vi "HighlandTester.vi"() -> ()   [LabVIEW 2013]
uses:
  <vilib>/Instr/_visa.llb/VISA Configure Serial Port (Instr).vi
  AlicatPC/AlicatPC.lvclass
panel:
  out "PULSE":bool
  out "return count":u32
  out "read buffer":string
  out "auto queue commands response":string
  out "error out":errorcluster
  in  "command":string="TLEVEL 1.25; TLEVEL; TRIG POS"
  out "response":string
  in  "VISA resource name":refnum<visa-resource-name>
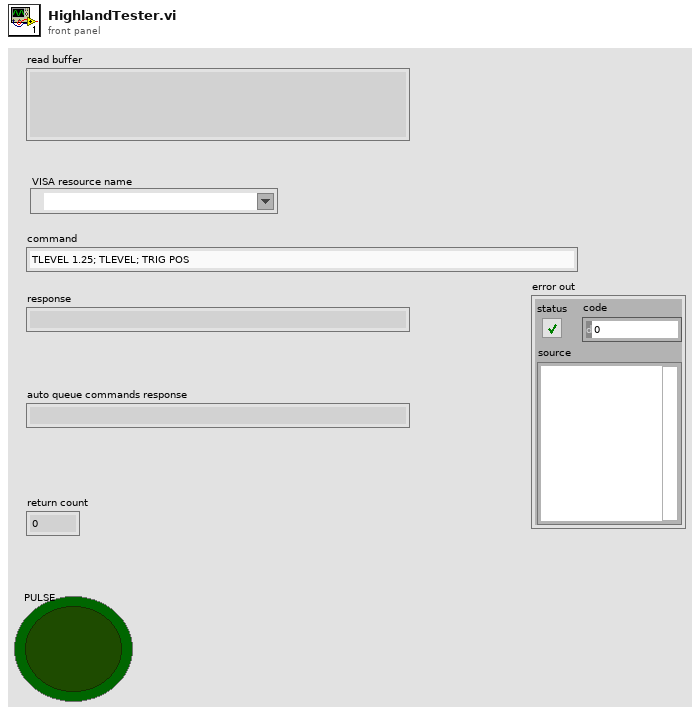
[diagram p1: front panel]
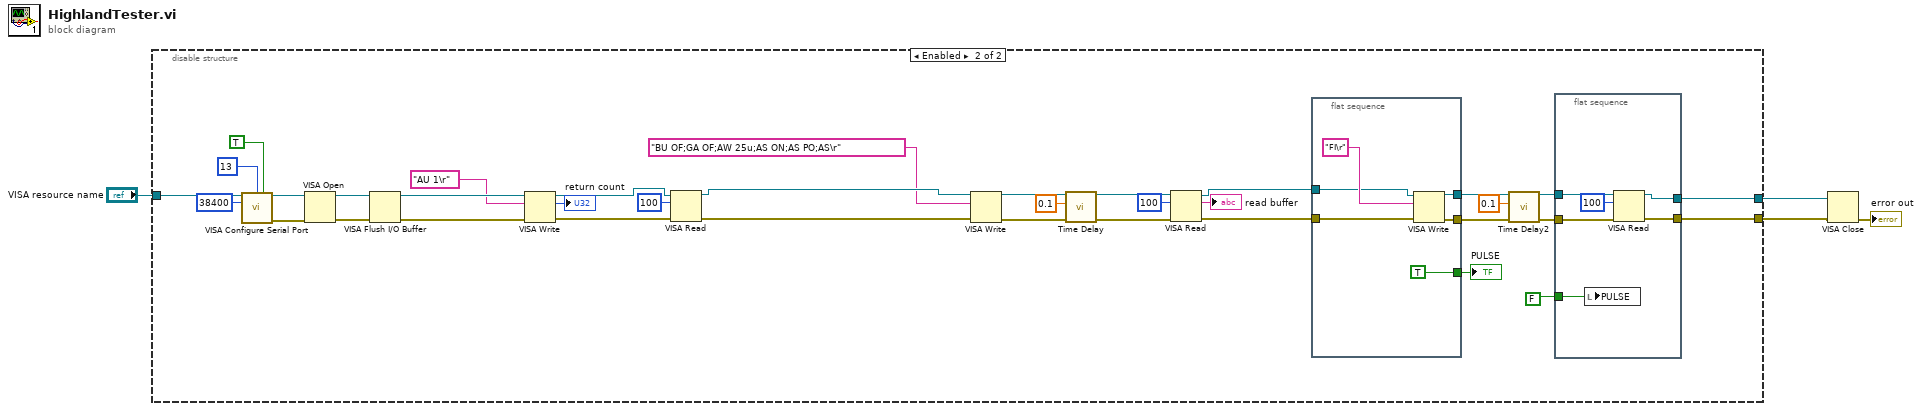
[diagram p0: block diagram]
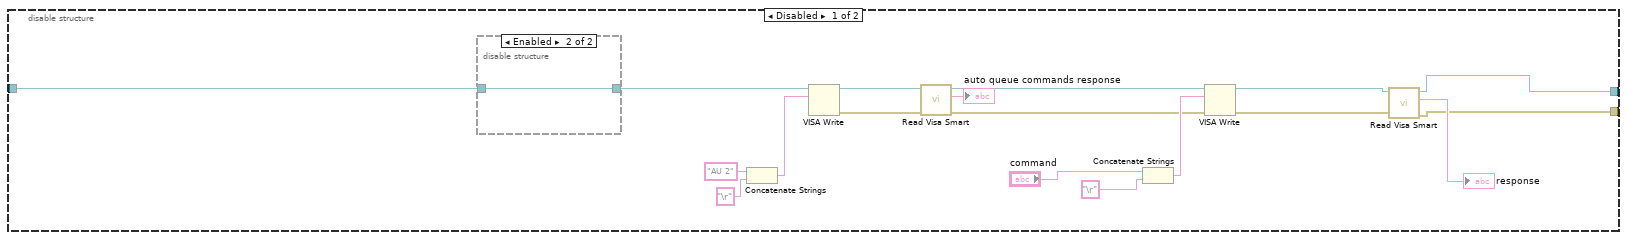
[diagram p2: hidden frame]
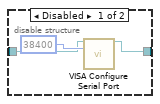
[diagram p3: hidden frame]
diagram:
  n1 = disable-structure shown="Enabled" {
    disable-tunnel: "VISA resource name" -> [w17 w54]
    disable-tunnel: [w16 w30] -> w3
    disable-tunnel: [w5 w29] -> w1
    frame Disabled {
      n2 = disable-structure shown="Enabled" {
        disable-tunnel: w17 -> [w24 w26]
        disable-tunnel: [w23 w26] -> w11
        frame Disabled {
          n3 = call-poly "VISA Configure Serial Port"("VISA resource name"=w24, "baud rate (9600)"=u32 38400) -> ("VISA resource name out"=w23:refnum<visa-resource-name>)  [unwired: 12 in, 1 out]
        }
        frame Enabled {
        }
      }
      n4 = Concatenate Strings("AU 2" ("string"), "\r") -> (w12:string)
      n5 = VISA Write(VISA resource name=w11, write buffer=w12) -> (VISA resource name out=w13:refnum<visa-resource-name>, error out=w14:errorcluster)  [unwired: 1 in, 1 out]
      n6 = call "Read Visa Smart.vi"("error in (no error)"=w14, "VISA Refnum in"=w13) -> ("error out"=w9:errorcluster, "String"=→"auto queue commands response":string, "VISA Refnum out"=w8:refnum<visa-resource-name>)  [unwired: 7 in]
      n7 = Concatenate Strings("command", "\r") -> (w20:string)
      n8 = VISA Write(VISA resource name=w8, write buffer=w20, error in (no error)=w9) -> (VISA resource name out=w19:refnum<visa-resource-name>, error out=w15:errorcluster)  [unwired: 1 out]
      n9 = call "Read Visa Smart.vi"("error in (no error)"=w15, "VISA Refnum in"=w19) -> ("error out"=w5:errorcluster, "String"=→"response":string, "VISA Refnum out"=w16:refnum<visa-resource-name>)  [unwired: 7 in]
    }
    frame Enabled {
      n10 = call-poly "VISA Configure Serial Port"("VISA resource name"=w54, "termination char\n(0xA = '\\n' = LF)"=u8 13 ("termination char\n(0xA = '\\n' = LF)"), "Enable Termination\nChar (T)"=TRUE ("Enable Termination\nChar (T)"), "baud rate (9600)"=u32 38400) -> ("VISA resource name out"=w53:refnum<visa-resource-name>, "error out"=w52:errorcluster)  [unwired: 10 in]
      n11 = VISA Open(error in (no error)=w52, VISA resource name=w53) -> (VISA resource name=w43:refnum<visa-resource-name>, error out=w41:errorcluster)  [unwired: 3 in]
      n12 = VISA Flush I/O Buffer(VISA resource name=w43, error in (no error)=w41) -> (VISA resource name out=w42:refnum<visa-resource-name>, error out=w40:errorcluster)  [unwired: 1 in]
      n13 = VISA Write(VISA resource name=w42, write buffer="AU 1\r", error in (no error)=w40) -> (VISA resource name out=w46:refnum<visa-resource-name>, return count=→"return count":u32, error out=w47:errorcluster)
      n14 = VISA Read(VISA resource name=w46, byte count=u32 100, error in (no error)=w47) -> (VISA resource name out=w45:refnum<visa-resource-name>, error out=w44:errorcluster)  [unwired: 2 out]
      n15 = VISA Write(VISA resource name=w45, write buffer="BU OF;GA OF;AW 25u;AS ON;AS PO;AS\r", error in (no error)=w44) -> (VISA resource name out=w60:refnum<visa-resource-name>, error out=w59:errorcluster)  [unwired: 1 out]
      n16 = call "Time Delay"("error in (no error)"=w59, "Delay Time (s)"=0.1) -> ("error out"=w56:errorcluster)  [unwired: 9 in]
      n17 = VISA Read(VISA resource name=w60, byte count=u32 100, error in (no error)=w56) -> (VISA resource name out=w31:refnum<visa-resource-name>, read buffer=→"read buffer":string, error out=w32:errorcluster)  [unwired: 1 out]
      n18 = flat-sequence {
        tunnel: [w71] -> w34
        tunnel: [w70] -> w33
        tunnel: w32 -> [w69]
        tunnel: w31 -> [w68]
        tunnel: [TRUE] -> w28
        frame #0 {
          n19 = VISA Write(VISA resource name=w68, write buffer="FI\r", error in (no error)=w69) -> (VISA resource name out=w70:refnum<visa-resource-name>, error out=w71:errorcluster)  [unwired: 1 out]
        }
      }
      n20 = call "Time Delay2"("error in (no error)"=w34, "Delay Time (s)"=0.1) -> ("error out"=w35:errorcluster)  [unwired: 9 in]
      n21 = flat-sequence {
        tunnel: w35 -> [w66]
        tunnel: w33 -> [w64]
        tunnel: [w63] -> w30
        tunnel: [w62] -> w29
        tunnel: FALSE -> [w61]
        frame #0 {
          n22 = local write "PULSE"(w61) -> ()
          n23 = VISA Read(VISA resource name=w64, byte count=u32 100, error in (no error)=w66) -> (VISA resource name out=w63:refnum<visa-resource-name>, error out=w62:errorcluster)  [unwired: 2 out]
        }
      }
      "PULSE" <- w28
    }
  }
  n24 = VISA Close(VISA resource name=w3, error in (no error)=w1) -> (error out=→"error out":errorcluster)
